vi "Scripting Main.vi"() -> ()   [LabVIEW 2019]
panel:
  in  "Insert BD into subpannel":bool
  in  "Insert FB into Sub Panel":bool
  in  "Set Settings":bool
  in  "Close FP":bool
  in  "Pane Color":u32(colorbox)
  in  "Control Settings":T1={"Text Color"=0, "BG Color"=0, "Label.Font:Name"="Didactic Gotic", "Font:Size"=5, "Label.Font:Bold"=FALSE} {"Font:Size" min=5 max=30 scale=0.0..30.0}
  in  "Open BD":bool
  in  "Open FP":bool
  in  "VIs in Project":i32(listbox)
  in  "Get All VIS Names":bool
  in  "Projects":u16(ring) items=["To test Scripting.lvproj"]
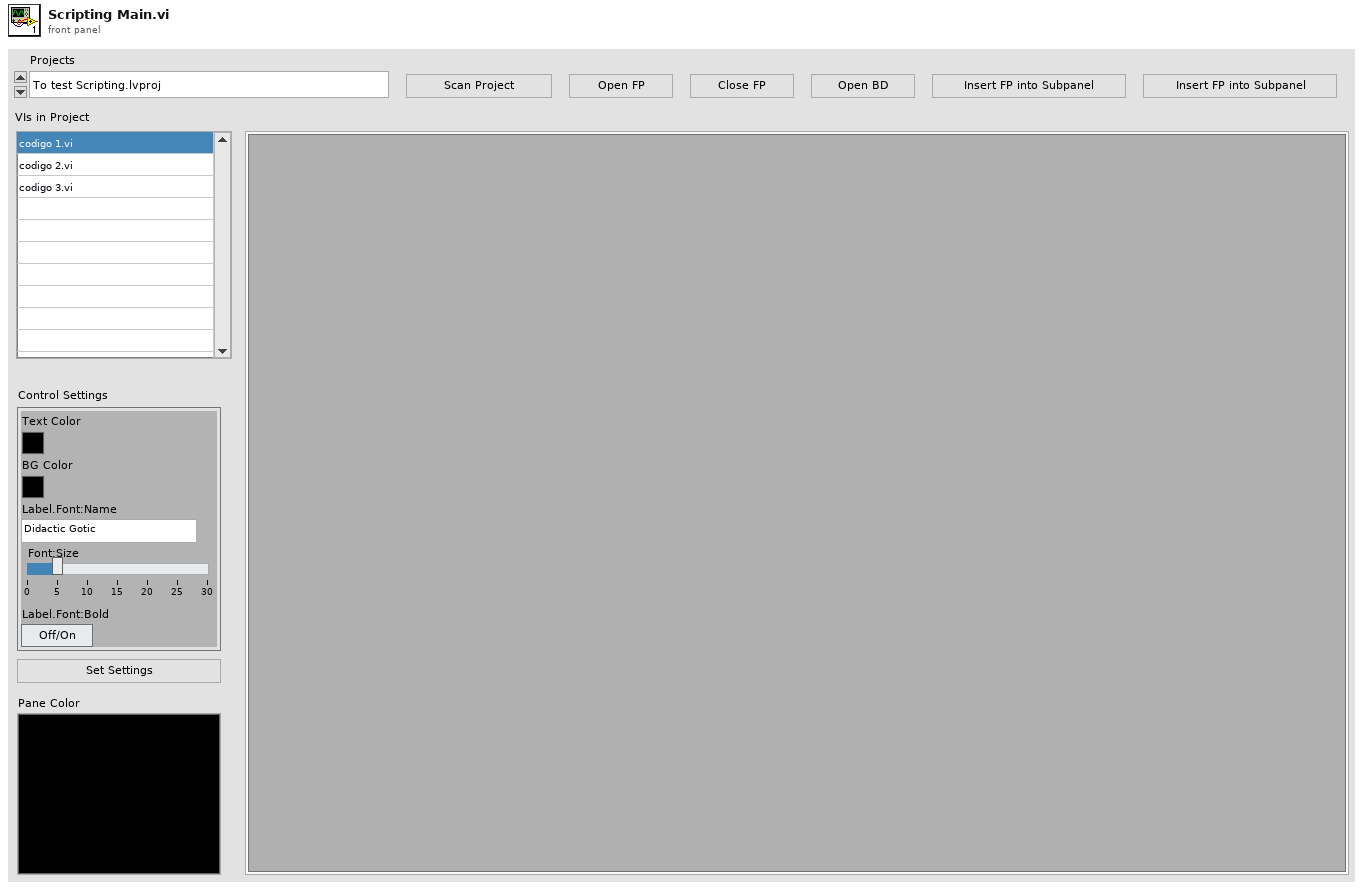
[diagram p1: front panel]
types:
  T1 = cluster{"Text Color":u32, "BG Color":u32, "Label.Font:Name":string, "Font:Size":u32, "Label.Font:Bold":bool}
  T2 = enum32{"Invalid", "Standard", "Closed", "Hidden", "Minimized", "Maximized"}
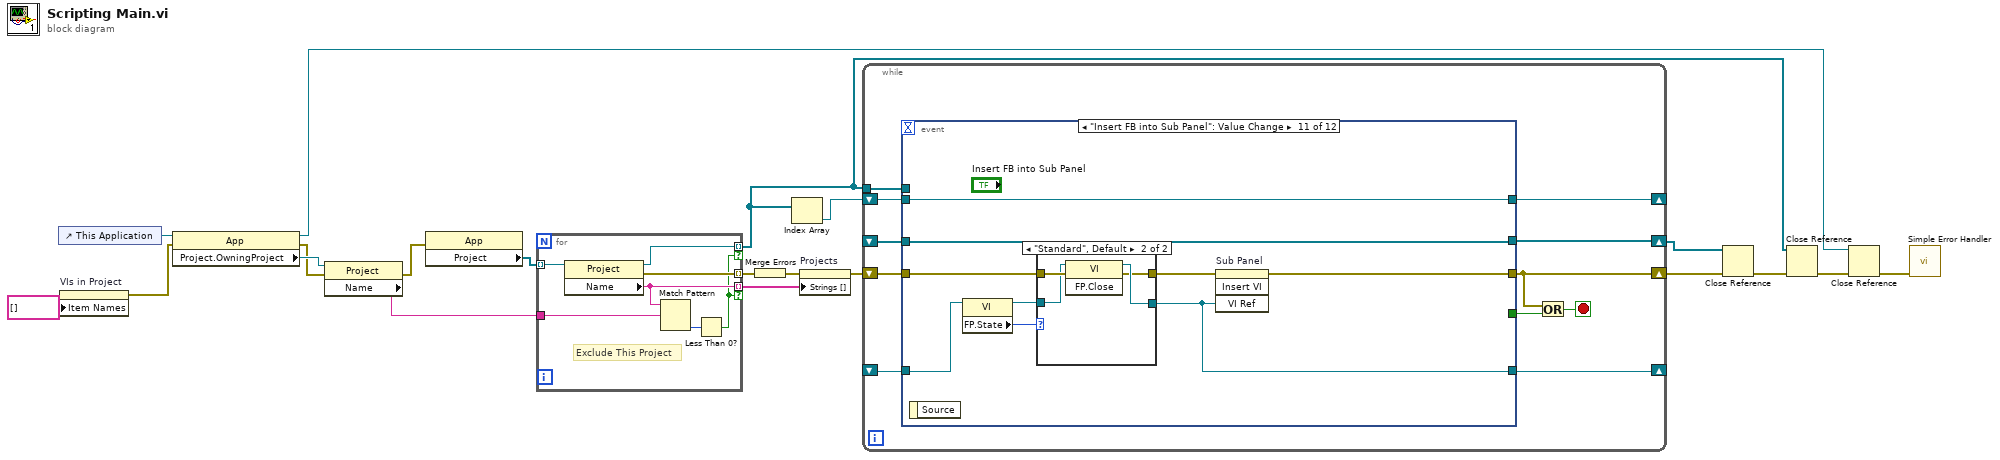
[diagram p0: block diagram]
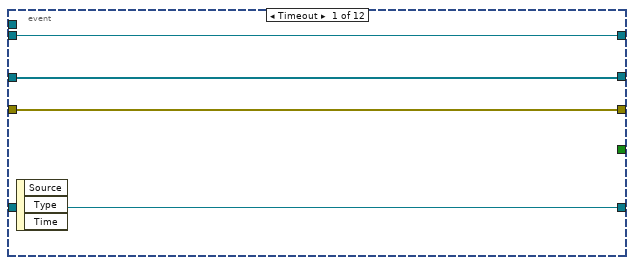
[diagram p2: hidden frame]
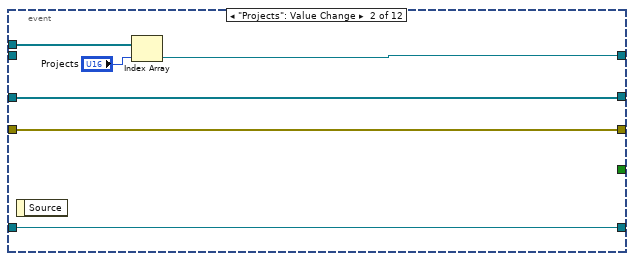
[diagram p3: hidden frame]
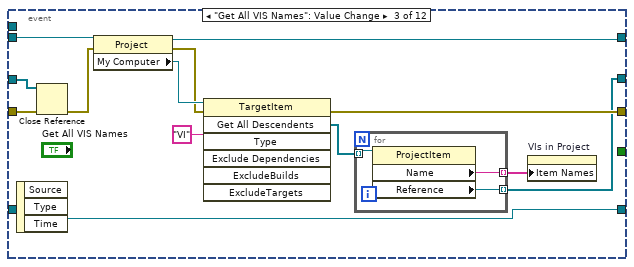
[diagram p4: hidden frame]
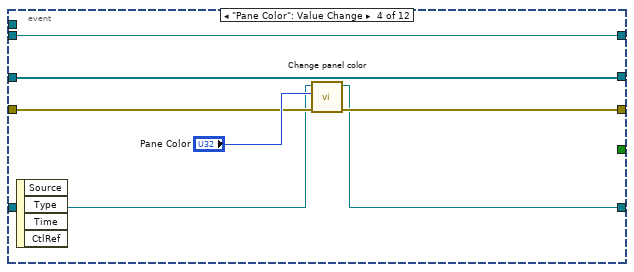
[diagram p5: hidden frame]
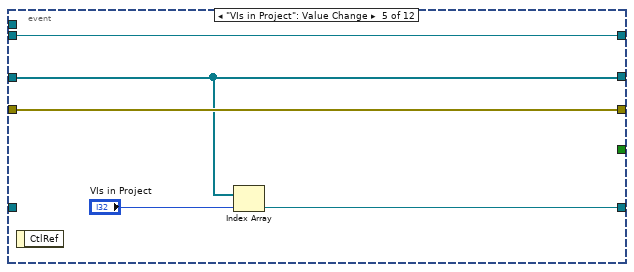
[diagram p6: hidden frame]
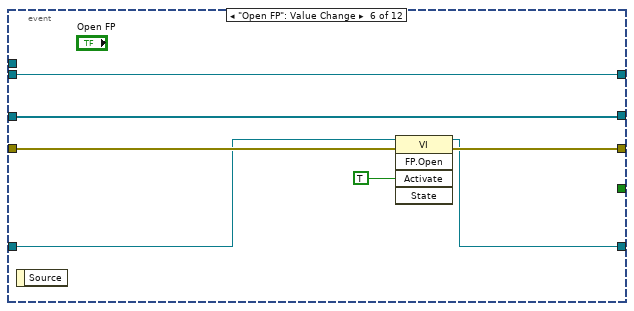
[diagram p7: hidden frame]
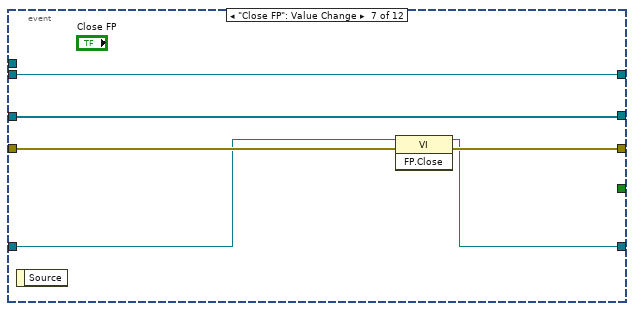
[diagram p8: hidden frame]
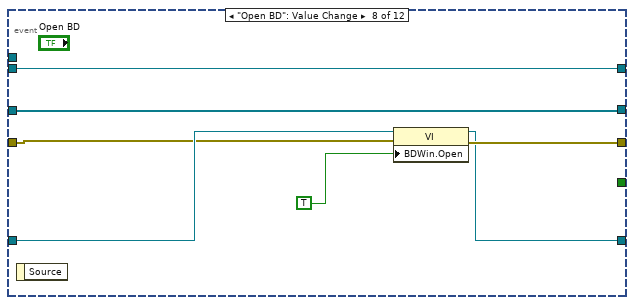
[diagram p9: hidden frame]
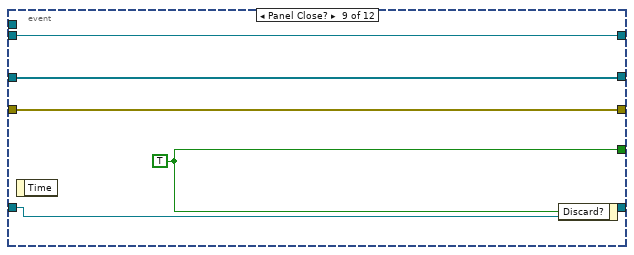
[diagram p10: hidden frame]
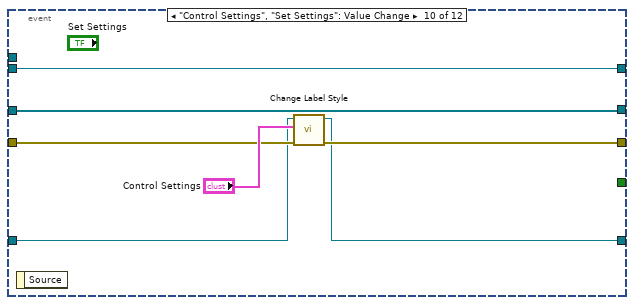
[diagram p11: hidden frame]
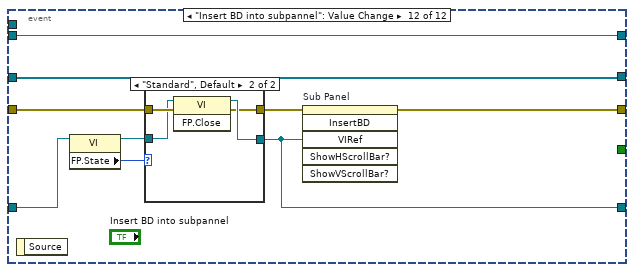
[diagram p13: hidden frame]
diagram:
  n1 = control-ref of="This Application"() -> (w19:refnum<vi>)
  n2 = property on="VIs in Project" class="LstBox (strict)"("Item Names"=string[] [] ("Strings []")) -> (error out=w2:errorcluster)  [unwired: 2 in, 1 out]
  n3 = property class="App"(reference=w19, error in=w2) -> (reference out=w8:refnum<vi>, error out=w7:errorcluster, "Project.OwningProject"=w18:refnum<vi>)
  n4 = property class="Project"(reference=w18, error in=w7) -> (error out=w6:errorcluster, "Name"=w17:string)  [unwired: 1 out]
  n5 = property class="App"(error in=w6) -> ("Project"=w15:refnum<vi>[])  [unwired: 1 in, 2 out]
  n6 = for {
    tunnel: w15 -> [w23] mode=indexing
    tunnel: [w26] -> w16 mode=indexing if=w21
    tunnel: w17 -> [w25]
    tunnel: [w27] -> w20 mode=indexing
    tunnel: [w22] -> w4 mode=indexing if=w21
    # "Exclude This Project"
    n7 = property class="Project"(reference=w23) -> (reference out=w22:refnum<vi>, error out=w27:errorcluster, "Name"=w26:string)  [unwired: 1 in]
    n8 = Match Pattern(string=w26, regular expression=w25) -> (offset past match=w24:i32)  [unwired: 1 in, 3 out]
    n9 = Less Than 0?(x=w24) -> (x < 0?=w21:bool)
  }
  n10 = Merge Errors(w20) -> (w14:errorcluster)
  n11 = Index Array(array=w4) -> (element=w3:refnum<vi>)  [unwired: 1 in]
  n12 = property on="Projects" class="Ring (strict)"(error in=w14, "Strings []"=w16) -> (error out=w13:errorcluster)  [unwired: 1 in, 1 out]
  n13 = while {
    tunnel: w4 -> [w38]
    shift-right: [w35] -> w11
    shift-left: w13 -> [w37]
    shift-right: [w33] -> _
    shift-left: w3 -> [w32]
    shift-right: [w31] -> w12
    shift-left: _ -> [w30]
    shift-right: [w29] -> _
    shift-left: _ -> [w28]
    stop <- w34 stop-if-true
    n14 = event shown="[10] \"Insert FB into Sub Panel\": Value Change" {
      selector: _ -> [_ _ _ _ _ _ _ _ _ _ _ _]
      dyn-events: _ -> [_ _ _ _ _ _ _ _ _ _ _ _]
      timeout: _ -> [_ _ _ _ _ _ _ _ _ _ _ _]
      tunnel: w38 -> [_ w48 _ _ _ _ _ _ _ _ _ _]
      tunnel: w37 -> [w42 w46 w50 w68 w76 w80 w87 w90 w101 w105 w112 w127]
      tunnel: [w42 w46 w56 w67 w76 w79 w86 w93 w101 w104 w113 w128] -> w35
      tunnel: [_ _ _ _ _ _ _ _ w100 _ _ _] -> w36
      tunnel: [w41 w45 w58 w71 w75 w83 w89 w96 w99 w108 w117 w132] -> w33
      tunnel: w32 -> [w41 _ w61 w71 w75 w83 w89 w96 w99 w108 w117 w132]
      tunnel: [w40 w44 w52 w70 w74 w82 w88 w95 w98 w107 w116 w131] -> w31
      tunnel: w30 -> [w40 w44 w51 w70 w74 w82 w88 w95 w98 w107 w116 w131]
      tunnel: [w39 w43 w53 w65 w72 w77 w84 w92 w97 w102 w115 w130] -> w29
      tunnel: w28 -> [w39 w43 w53 w66 _ w78 w85 w91 w97 w103 w111 w126]
      event Timeout {
        n15 = event-data() -> ()  [unwired: 1 in, 3 out]
      }
      event "Projects": Value Change {
        n16 = event-data() -> ()  [unwired: 1 in, 1 out]
        n17 = Index Array(array=w48, index="Projects") -> (element=w45:refnum<vi>)
      }
      event "Get All VIS Names": Value Change {
        n18 = event-data() -> ()  [unwired: 1 in, 3 out]
        n19 = Close Reference(reference=w51, error in (no error)=w50) -> (error out=w49:errorcluster)
        n20 = property class="Project"(reference=w61, error in=w49) -> (reference out=w58:refnum<vi>, error out=w59:errorcluster, "My Computer"=w60:refnum<vi>)
        n21 = invoke class="TargetItem" method="Get All Descendents"(reference=w60, error in=w59, "Type"="VI") -> (error out=w56:errorcluster, "All Descendents"=w54:refnum<vi>[])  [unwired: 4 in, 5 out]
        n22 = for {
          tunnel: w54 -> [w64] mode=indexing
          tunnel: [w63] -> w55 mode=indexing
          tunnel: [w62] -> w52 mode=indexing
          n23 = property class="ProjectItem"(reference=w64) -> ("Name"=w63:string, "Reference"=w62:refnum<vi>)  [unwired: 1 in, 2 out]
        }
        n24 = property on="VIs in Project" class="LstBox (strict)"("Item Names"=w55) -> ()  [unwired: 2 in, 2 out]
      }
      event "Pane Color": Value Change {
        n25 = event-data() -> ()  [unwired: 1 in, 4 out]
        n26 = call "Change panel color.vi"("error in"=w68, "Pane Color"="Pane Color", "VI in"=w66) -> ("error out"=w67:errorcluster, "VI out"=w65:refnum<vi>)  [unwired: 7 in]
      }
      event "VIs in Project": Value Change {
        n27 = event-data() -> ()  [unwired: 1 in, 1 out]
        n28 = Index Array(array=w74, index="VIs in Project") -> (element=w72:refnum<vi>)
      }
      event "Open FP": Value Change {
        n29 = event-data() -> ()  [unwired: 1 in, 1 out]
        n30 = invoke class="VI" method="FP.Open"(reference=w78, error in=w80, "Activate"=TRUE ("Activate?")) -> (reference out=w77:refnum<vi>, error out=w79:errorcluster)  [unwired: 2 in, 3 out]
      }
      event "Close FP": Value Change {
        n31 = event-data() -> ()  [unwired: 1 in, 1 out]
        n32 = invoke class="VI" method="FP.Close"(reference=w85, error in=w87) -> (reference out=w84:refnum<vi>, error out=w86:errorcluster)  [unwired: 1 in, 1 out]
      }
      event "Open BD": Value Change {
        n33 = event-data() -> ()  [unwired: 1 in, 1 out]
        n34 = property on="Property Node" class="VI"(reference=w91, error in=w90, "BDWin.Open"=TRUE ("Block Diagram Window:Open")) -> (reference out=w92:refnum<vi>, error out=w93:errorcluster)
      }
      event Panel Close? {
        w100 = TRUE ("Discard?")
        n35 = event-data() -> ()  [unwired: 1 in, 1 out]
        n36 = event-data("Discard?"=w100) -> ()  [unwired: 1 in, 1 out]
      }
      event "Control Settings", "Set Settings": Value Change {
        n37 = event-data() -> ()  [unwired: 1 in, 1 out]
        n38 = call "Change Label Style.vi"("error in"=w105, "Settinngs"="Control Settings", "VI in"=w103) -> ("error out"=w104:errorcluster, "VI out"=w102:refnum<vi>)  [unwired: 7 in]
      }
      event "Insert FB into Sub Panel": Value Change {
        n39 = event-data() -> ()  [unwired: 1 in, 1 out]
        n40 = property class="VI"(reference=w111) -> (reference out=w109:refnum<vi>, "FP.State"=w110:T2)  [unwired: 1 in, 1 out]
        n41 = case shown="\"Standard\", Default" w110 {
          tunnel: [w118 w123] -> w115
          tunnel: [w119 w122] -> w114
          tunnel: w112 -> [w119 w121]
          tunnel: w109 -> [w118 w120]
          frame "Invalid", "Closed" {
          }
          frame "Standard", Default {
            n42 = invoke class="VI" method="FP.Close"(reference=w120, error in=w121) -> (reference out=w123:refnum<vi>, error out=w122:errorcluster)  [unwired: 1 in, 1 out]
          }
        }
        n43 = invoke on="Sub Panel" class="SubPnl" method="Insert VI"(error in=w114, "VI Ref"=w115) -> (error out=w113:errorcluster)  [unwired: 2 in, 3 out]
      }
      event "Insert BD into subpannel": Value Change {
        n44 = event-data() -> ()  [unwired: 1 in, 1 out]
        n45 = property class="VI"(reference=w126) -> (reference out=w124:refnum<vi>, "FP.State"=w125:T2)  [unwired: 1 in, 1 out]
        n46 = case shown="\"Standard\", Default" w125 {
          tunnel: [w133 w138] -> w130
          tunnel: [w134 w137] -> w129
          tunnel: w127 -> [w134 w136]
          tunnel: w124 -> [w133 w135]
          frame "Invalid", "Closed" {
          }
          frame "Standard", Default {
            n47 = invoke class="VI" method="FP.Close"(reference=w135, error in=w136) -> (reference out=w138:refnum<vi>, error out=w137:errorcluster)  [unwired: 1 in, 1 out]
          }
        }
        n48 = invoke on="Sub Panel" class="SubPnl" method="InsertBD"(error in=w129, "VIRef"=w130) -> (error out=w128:errorcluster)  [unwired: 4 in, 5 out]
      }
    }
    n49 = Or(x=w35, y=w36) -> (x .or. y?=w34:bool)
  }
  n50 = Close Reference(reference=w12, error in (no error)=w11) -> (error out=w10:errorcluster)
  n51 = Close Reference(reference=w4, error in (no error)=w10) -> (error out=w9:errorcluster)
  n52 = Close Reference(reference=w8, error in (no error)=w9) -> (error out=w5:errorcluster)
  n53 = call <vilib>:"Simple Error Handler.vi"("error in (no error)"=w5) -> ()  [unwired: 4 in, 5 out]
